vi "send shape.vi"(8 "error in (no error)":errorcluster, 10 "1x160 Voltage Map":dbl[](array[numeric]), 11 "BMC in":refnum<class "BMC.lvclass">) -> (0 "error out":errorcluster, 3 "BMC out":refnum<class "BMC.lvclass">)   [LabVIEW 2012, in "BMC.lvclass"]
uses:
  BMC.lvclass
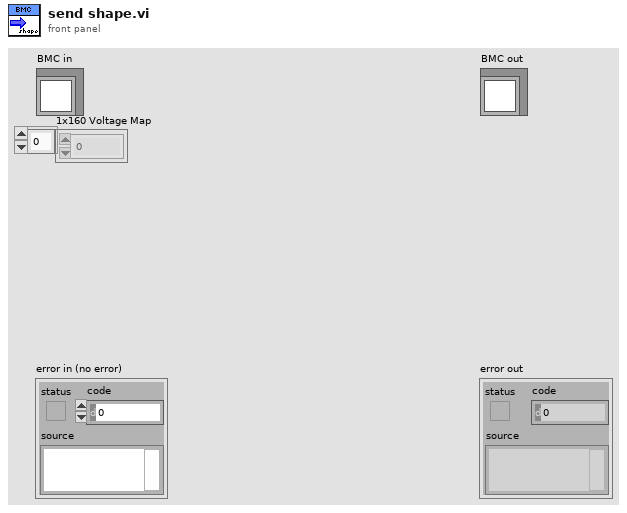
[diagram p1: front panel]
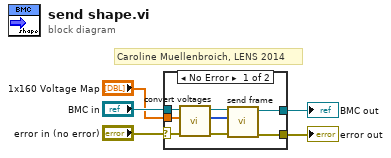
[diagram p0: block diagram]
diagram:
  # "Caroline Muellenbroich, LENS 2014"
  n1 = case shown="No Error" "error in (no error)" {
    selector: "error in (no error)" -> [w13 w15]
    tunnel: [w11 w15] -> w4
    tunnel: [w10 w14] -> w2
    tunnel: "BMC in" -> [w8 w14]
    tunnel: "1x160 Voltage Map" -> [w6 _]
    frame No Error {
      n2 = call-dynamic "convert voltages.vi"("error in (no error)"=w13, "1x160 Voltage Map"=w6, "BMC in"=w8) -> ("error out"=w12:errorcluster, "Voltage array out"=w7:u16[], "BMC out"=w9:refnum<class "BMC.lvclass">)  [unwired: 6 in]
      n3 = call-dynamic "send frame.vi"("error in (no error)"=w12, "Voltage array"=w7, "BMC in"=w9) -> ("error out"=w11:errorcluster, "BMC out"=w10:refnum<class "BMC.lvclass">)  [unwired: 7 in]
    }
    frame Error {
    }
  }
  "error out" <- w4
  "BMC out" <- w2
